vi "Znorm_d4app_fields.vi"(8 "error in (no error)":errorcluster, 9 "acceptance angle":dbl, 11 "Zn":dbl) -> (0 "error out":errorcluster, 1 "E field":string, 3 "Phase Field":string)   [LabVIEW 2017]
panel:
  out "d4app":dbl
  out "min val":dbl
  out "u32 number":u32
  out "d4app bool array":bool[](array[boolean])
  out "d4appmin":dbl
  out "znorm_int_string":string
  out "znorm_objective":string
  out "check bool array":bool[](array[boolean])
  out "u16 version":u16
  out "fixed-point":fxp<+,16,0>
  out "bool array":bool[](array[boolean])
  out "znorm/10000":dbl
  in  "znormscale":dbl
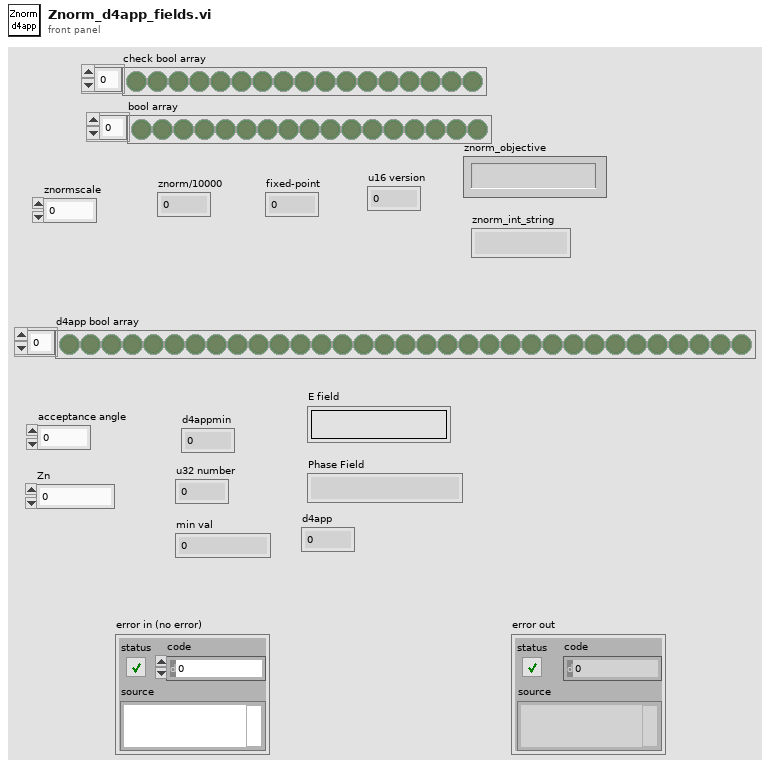
[diagram p1: front panel]
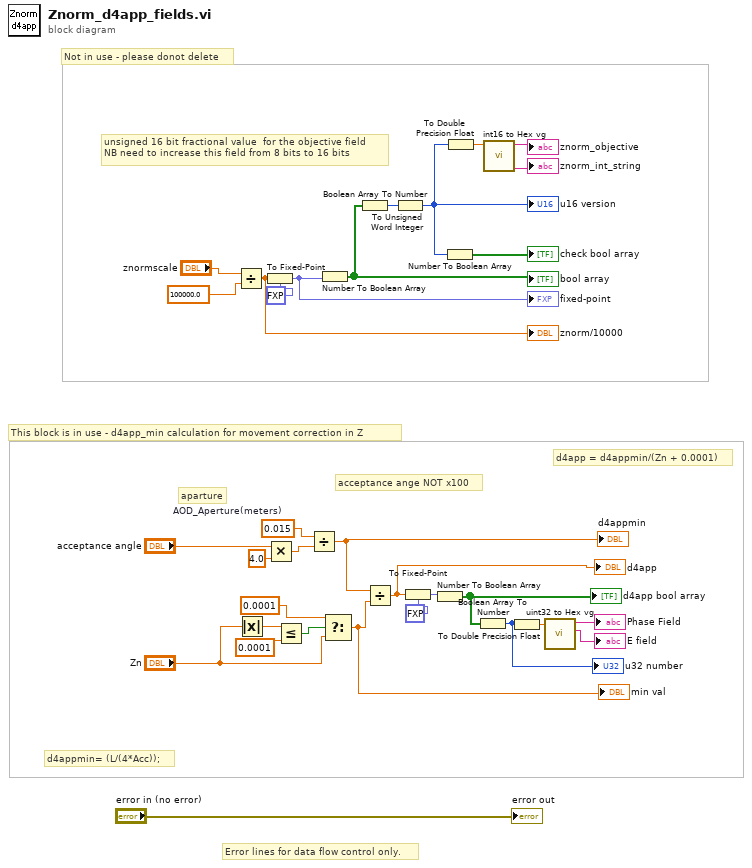
[diagram p0: block diagram]
diagram:
  w19 = 0.015  # AOD_Aperture(meters)
  # "Error lines for data flow control only."
  # "Not in use - please donot delete"
  # "This block is in use - d4app_min calculation for movement correction in Z"
  # "acceptance ange NOT x100"
  # "aparture"
  # "unsigned 16 bit fractional value  for the objective field\nNB need to increase this field from 8 bits to 16 bits"
  # "d4app = d4appmin/(Zn + 0.0001)"
  # "d4appmin= (L/(4*Acc));"
  n1 = Divide(x="znormscale", y=100000.0) -> (x/y=w30:dbl)
  "znorm/10000" <- w30
  n2 = Absolute Value(x="Zn") -> (abs(x)=w10:dbl)
  n3 = To Fixed-Point(fixed-point type=fxp<+,16,0> 0.0, number=w30) -> (fixed-point=w29:fxp<+,16,0>)
  "fixed-point" <- w29
  n4 = Multiply(x="acceptance angle", y=4.0) -> (x*y=w20:dbl)
  n5 = Less Or Equal?(x=w10, y=0.0001 ("x")) -> (x <= y?=w8:bool)
  n6 = Divide(x=w19, y=w20) -> (x/y=w5:dbl)
  "d4appmin" <- w5
  n7 = Number To Boolean Array(number=w29) -> (Boolean array=w4:bool[])
  "bool array" <- w4
  n8 = Select(t=0.0001 ("x"), s=w8, f="Zn") -> (s? t:f=w6:dbl)
  "min val" <- w6
  n9 = Boolean Array To Number(Boolean array=w4) -> (number=w26:u32)
  n10 = Divide(x=w5, y=w6) -> (x/y=w17:dbl)
  "d4app" <- w17
  n11 = To Unsigned Word Integer(number=w26) -> (unsigned 16bit integer=w15:u16)
  "u16 version" <- w15
  n12 = To Fixed-Point(fixed-point type=fxp<+/-,32,16> 0.0, number=w17) -> (fixed-point=w16:fxp<+/-,32,16>)
  n13 = Number To Boolean Array(number=w16) -> (Boolean array=w14:bool[])
  "d4app bool array" <- w14
  n14 = Number To Boolean Array(number=w15) -> (Boolean array=→"check bool array":bool[])
  n15 = To Double Precision Float(number=w15) -> (double precision float=w24:dbl)
  n16 = Boolean Array To Number(Boolean array=w14) -> (number=w13:u32)
  "u32 number" <- w13
  n17 = call "int16 to Hex vg.vi"("number"=w24) -> ("hex integer string"=→"znorm_int_string":string, "Hex string"=→"znorm_objective":string)  [unwired: 9 in]
  n18 = To Double Precision Float(number=w13) -> (double precision float=w12:dbl)
  n19 = call "uint32 to Hex vg.vi"("number"=w12) -> ("[31:16]"=→"E field":string, "[15:0]"=→"Phase Field":string)  [unwired: 8 in, 1 out]
  "error out" <- "error in (no error)"
